vi "Get UIAs prefixes.vi"(11 "DualScreenV in":refnum<class "DualScreenV.lvclass">) -> (2 "2nd UIA prefix":string, 3 "1st UIA prefix":string)   [LabVIEW 2020, in "DualScreenV.lvlib" / "DualScreenV.lvclass"]
uses:
  DualScreenV.lvclass
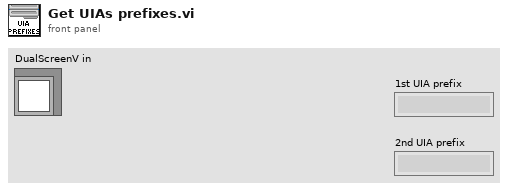
[diagram p1: front panel]
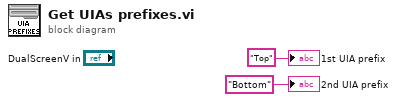
[diagram p0: block diagram]
diagram:
  "1st UIA prefix" <- "Top" ("String")
  "2nd UIA prefix" <- "Bottom" ("String")
